vi "Perform Measurement.vi"(6 "wait for reply (T)":bool=TRUE, 8 "error in (no error)":errorcluster, 10 "read_source":T2(ring)) -> (0 "error out":errorcluster, 1 "timed out?":bool, 2 "Reply Payload":T1 {"module_id" items=["thcd"=301]})   [LabVIEW 2020, in "1039_mod.lvlib"]
doc: "_____\nCreated using Delacor QMH Event Scripter 4.2.1.88."
uses:
  1039_mod.lvlib
  Perform Measurement (Reply Payload)--cluster.ctl
  Perform Measurement Argument--cluster.ctl
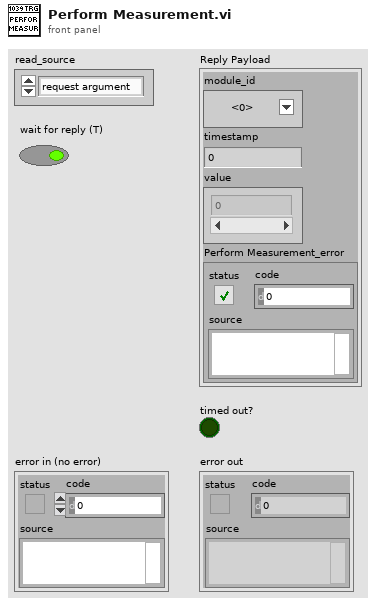
[diagram p1: front panel]
types:
  T1 = typedef "1039_mod.lvlib/Perform Measurement (Reply Payload)--cluster.ctl" = cluster{"module_id":u16, "timestamp":dbl, "value":dbl[], "Perform Measurement_error":errorcluster}
  T2 = enum16{"request argument", "configuration file", "module setting"}
  T3 = typedef "1039_mod.lvlib/Perform Measurement Argument--cluster.ctl" = cluster{"read_source":enum16{"request argument", "configuration file", "module setting"}, "Wait Notifier":refnum<notifier>, "wait for reply":bool}
  T4 = typedef "1039_mod.lvlib/Request Events--cluster.ctl" = cluster{"Stop Module":refnum<user-event>, "Show Panel":refnum<user-event>, "Hide Panel":refnum<user-event>, "Get Module Execution Status":refnum<user-event>, "Show Diagram":refnum<user-event>, "Initialize Communication":refnum<user-event>, "Initialize Instrument":refnum<user-event>, "Configure Instrument":refnum<user-event>, "Perform Measurement":refnum<user-event>}
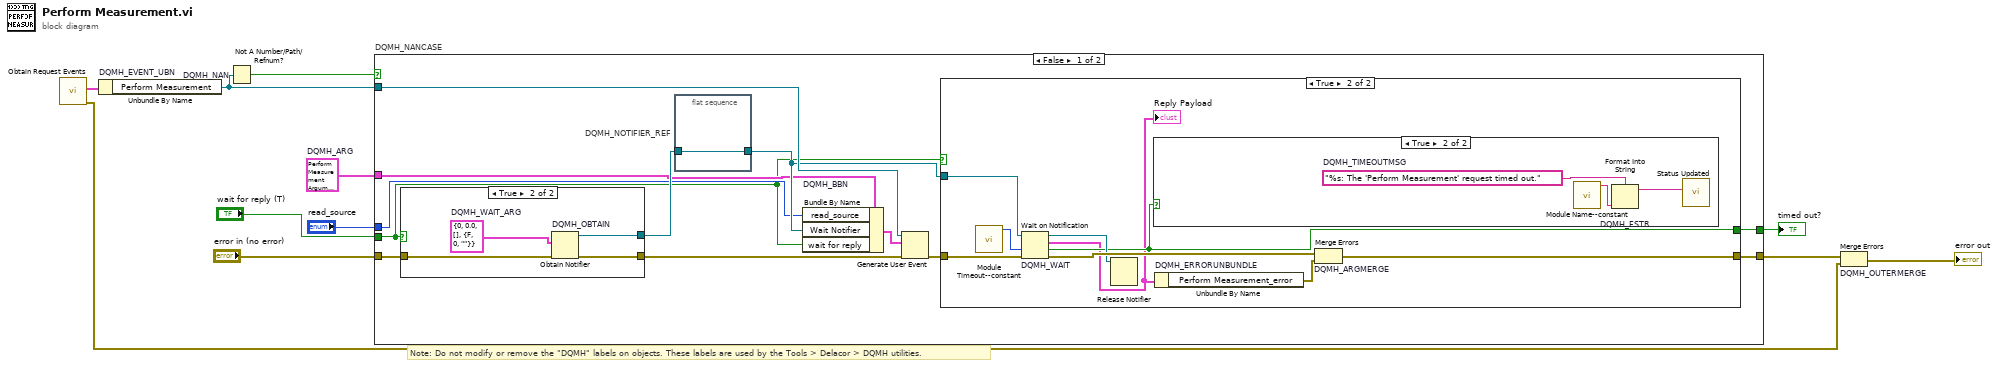
[diagram p0: block diagram]
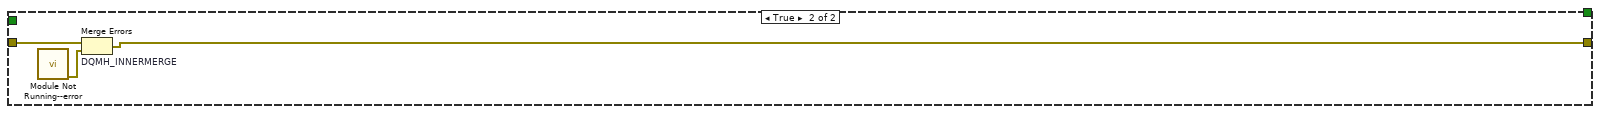
[diagram p5: hidden frame]
diagram:
  w5 = T3 {"read_source"=enum."request argument", "Wait Notifier"=refnum, "wait for reply"=FALSE}  # DQMH_ARG
  # "Note: Do not modify or remove the \"DQMH\" labels on objects. These labels are used by the Tools > Delacor > DQMH utilities."
  n1 = call "Obtain Request Events.vi"() -> ("error out"=w2:errorcluster, "1039_mod Request Events"=w1:T4)  [unwired: 10 in]
  n2 = Unbundle By Name "DQMH_EVENT_UBN"(w1) -> ("Perform Measurement"=w9:refnum<user-event>)
  n3 = Not A Number/Path/Refnum? "DQMH_NAN"(number/path/refnum=w9) -> (NaN/Path/Refnum?=w8:bool)
  n4 = case "DQMH_NANCASE" shown="False" w8 {
    tunnel: "error in (no error)" -> [w23 w45]
    tunnel: w9 -> [w21 _]
    tunnel: [w18 w44] -> w6
    tunnel: [w19 _] -> w7
    tunnel: w5 -> [w14 _]
    tunnel: "read_source" -> [w13 _]
    tunnel: "wait for reply (T)" -> [w12 _]
    frame False {
      n5 = case shown="True" w12 {
        tunnel: w23 -> [w38 w42]
        tunnel: [w38 w41] -> w20
        tunnel: [_ w39] -> w16
        frame False {
        }
        frame True {
          w40 = T1 {"module_id"=0, "timestamp"=0.0, "value"=[], "Perform Measurement_error"={"status"=FALSE, "code"=0, "source"=""}}  # DQMH_WAIT_ARG
          n6 = Obtain Notifier "DQMH_OBTAIN"(notification data type=w40, error in (no error)=w42) -> (notifier out=w39:refnum<notifier>, error out=w41:errorcluster)  [unwired: 2 in, 1 out]
        }
      }
      n7 = flat-sequence "DQMH_NOTIFIER_REF" {
        tunnel: w16 -> [w24]
        tunnel: [w24] -> w15
        frame #0 {
        }
      }
      n8 = Bundle By Name "DQMH_BBN"(cluster=w14, "read_source"=w13, "Wait Notifier"=w15, "wait for reply"=w12) -> (w17:T3)
      n9 = Generate User Event(user event=w21, event data cluster=w17, error in=w20) -> (error out=w22:errorcluster)  [unwired: 1 in, 1 out]
      n10 = case shown="True" w12 {
        tunnel: w22 -> [w25 w34]
        tunnel: w15 -> [_ w32]
        tunnel: [_ w30] -> w19
        tunnel: [w25 w29] -> w18
        frame False {
        }
        frame True {
          n11 = call "Module Timeout--constant.vi"() -> ("Module Timeout"=w26:i32)  [unwired: 11 in]
          n12 = Wait on Notification "DQMH_WAIT"(notifier=w32, timeout in ms (-1)=w26, error in (no error)=w34) -> (notifier out=w31:refnum<notifier>, notification=w27:T1, timed out?=w30:bool, error out=w33:errorcluster)  [unwired: 1 in]
          "Reply Payload" <- w27
          n13 = Release Notifier(notifier=w31) -> ()  [unwired: 2 in, 3 out]
          n14 = case shown="True" w30 {
            frame False {
            }
            frame True {
              w37 = "%s: The 'Perform Measurement' request timed out."  # DQMH_TIMEOUTMSG
              n15 = call "Module Name--constant.vi"() -> ("Module Name"=w36:string)  [unwired: 11 in]
              n16 = Format Into String "DQMH_FSTR"(format string=w37, w36) -> (resulting string=w35:string)  [unwired: 2 in, 1 out]
              n17 = call "Status Updated.vi"("Status"=w35) -> ()  [unwired: 10 in, 1 out]
            }
          }
          n18 = Unbundle By Name "DQMH_ERRORUNBUNDLE"(w27) -> ("Perform Measurement_error"=w28:errorcluster)
          n19 = Merge Errors "DQMH_ARGMERGE"(w33, w28) -> (w29:errorcluster)
        }
      }
    }
    frame True {
      n20 = call "Module Not Running--error.vi"() -> ("error out"=w43:errorcluster)  [unwired: 11 in]
      n21 = Merge Errors "DQMH_INNERMERGE"(w45, w43) -> (w44:errorcluster)
    }
  }
  "timed out?" <- w7
  n22 = Merge Errors "DQMH_OUTERMERGE"(w6, w2) -> (→"error out":errorcluster)
